vi "Test Helper Loop waiting for Start.vi"(8 "error in (no error)":errorcluster, 11 "Helper Loop Test In":refnum<class "Helper Loop Test.lvclass">) -> (0 "error out":errorcluster, 3 "Helper Loop Test Out":refnum<class "Helper Loop Test.lvclass">)   [LabVIEW 2020, in "Helper Loop Test.lvclass"]
uses:
  Helper Loop Test.lvclass
  Mock Process/Mock Process.lvclass
  <vilib>/Asteme/LUnit/Test Case.lvclass
  Framework/Process/Process.lvclass
  Support/Framework Test Support.lvlib
  Support/Event Helpers/Event Helpers.lvlib
  C:/Users/anton/Documents/GitHub/Triarc-Framework/source/Framework/Process/Process.lvclass
  C:/Users/anton/Documents/GitHub/Triarc-Framework/source/Framework/Base/Base.lvclass
  C:/Users/anton/Documents/GitHub/Triarc-Framework/source/Framework/Configuration File/Configuration File.lvclass
  C:/Users/anton/Documents/GitHub/Triarc-Framework/source/Framework/Error Handler Interface/Error Handler Interface.lvclass
  C:/Users/anton/Documents/GitHub/Triarc-Framework/source/Framework Test/Mock Process/Mock Process.lvclass
  C:/Users/anton/Documents/GitHub/Triarc-Framework/source/Framework/Helper Loop/Helper Loop.lvclass
  C:/Program Files (x86)/National Instruments/LabVIEW 2020/vi.lib/Asteme/LUnit/Test Case.lvclass
  C:/Users/anton/Documents/GitHub/Triarc-Framework/source/Framework Test/Helper Loop Test/Helper Loop Test.lvclass
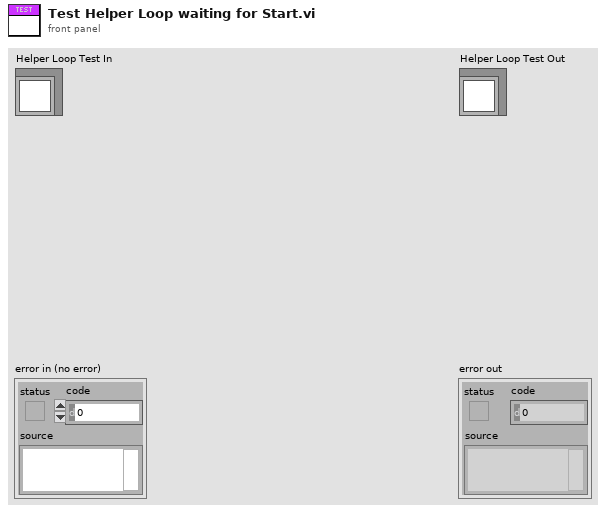
[diagram p1: front panel]
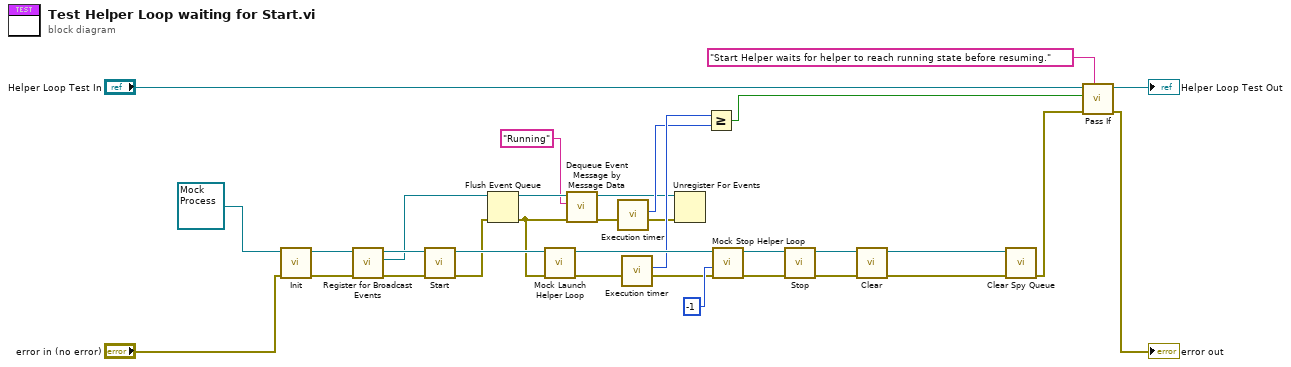
[diagram p0: block diagram]
diagram:
  n1 = call-dynamic "Init.vi"("error in (no error)"="error in (no error)", "Mock Process In"=refnum<class "Mock Process.lvclass"> refnum) -> ("error out"=w31:errorcluster, "Mock Process Out"=w32:refnum<class "Mock Process.lvclass">)  [unwired: 8 in]
  n2 = call-dynamic "Register for Broadcast Events.vi"("error in (no error)"=w31, "Process In"=w32) -> ("error out"=w29:errorcluster, "Event Registration Refnum"=w13:refnum<event-registration>, "Process Out"=w30:refnum<class "Mock Process.lvclass">)  [unwired: 7 in]
  n3 = call "Start.vi"("error in (no error)"=w29, "Process In"=w30) -> ("error out"=w11:errorcluster, "Process Out"=w28:refnum<class "Mock Process.lvclass">)  [unwired: 8 in]
  n4 = Flush Event Queue(0:w13, 3:w11) -> (8:w12:refnum<event-registration>, 11:w3:errorcluster)  [unwired: 4 in, 1 out]
  n5 = call "Mock Launch Helper Loop.vi"("error in (no error)"=w3, "Mock Process in"=w28) -> ("error out"=w9:errorcluster, "Mock Process out"=w27:refnum<class "Mock Process.lvclass">)  [unwired: 8 in]
  n6 = call "Dequeue Event Message by Message Data.vi"("error in (no error)"=w3, "Message Data"="Running", "Event Registration Refnum"=w12) -> ("error out"=w10:errorcluster, "Event Registration Refnum Out"=w4:refnum<event-registration>)  [unwired: 4 in, 3 out]
  n7 = call "Execution timer.vi"("error in (no error)"=w10) -> ("error out"=w5:errorcluster, "Current or Duration [ms]"=w6:u32)  [unwired: 9 in]
  n8 = call "Execution timer.vi"("error in (no error)"=w9) -> ("error out"=w8:errorcluster, "Current or Duration [ms]"=w7:u32)  [unwired: 9 in]
  n9 = Unregister For Events(event registration refnum=w4, error in=w5) -> ()  [unwired: 1 out]
  n10 = Greater Or Equal?(x=w7, y=w6) -> (x >= y?=w2:bool)
  n11 = call "Mock Stop Helper Loop.vi"("error in (no error)"=w8, "timeout in ms (-1)"=-1, "Mock Process in"=w27) -> ("error out"=w25:errorcluster, "Mock Process out"=w26:refnum<class "Mock Process.lvclass">)  [unwired: 6 in, 1 out]
  n12 = call "Stop.vi"("error in (no error)"=w25, "Process In"=w26) -> ("error out"=w23:errorcluster, "Process Out"=w24:refnum<class "Mock Process.lvclass">)  [unwired: 7 in, 1 out]
  n13 = call-dynamic "Clear.vi"("error in (no error)"=w23, "Mock Process In"=w24) -> ("error out"=w21:errorcluster, "Mock Process Out"=w22:refnum<class "Mock Process.lvclass">)  [unwired: 8 in]
  n14 = call-dynamic "Clear Spy Queue.vi"("error in (no error)"=w21, "Mock Process In"=w22) -> ("error out"=w17:errorcluster)  [unwired: 8 in, 1 out]
  n15 = call <vilib>:"Pass If.vi"("Description"="Start Helper waits for helper to reach running state before resuming.", "error in (no error)"=w17, "Pass?"=w2, "Test Case In"="Helper Loop Test In") -> ("error out"=→"error out":errorcluster, "Test Case Out"=→"Helper Loop Test Out":refnum<class "Helper Loop Test.lvclass">)  [unwired: 6 in]
